vi "SEA-9510 FPGA.vi"() -> ()   [LabVIEW 2019]
doc: "Copyright (c) 2015-2019 S.E.A. Datentechnik GmbH, Germany"
uses:
  <vilib>/rvi/Emulation/niFpgaSctlEmulationGetInTimedLoop.vi
  <vilib>/rvi/Emulation/niFpgaProcessEmulError.vi
  <vilib>/rvi/eio/common/nirviEmuTemplateMethod_errors.vi
  <vilib>/rvi/Emulation/niFpgaGetClockAttributes.vi
  <vilib>/rvi/Emulation/niFpgaEmulationReportErrorSimple.vi
  <vilib>/rvi/Emulation/niFpgaCriticalErrorInLSC.vi
  <vilib>/eio/EIOMethodNode/EIOMethodNode.xnode
  <vilib>/eio/EIONode/EIONode.xnode
panel:
  in  "Numeric 3":i16
  out "Numeric 2":i16
  in  "Boolean":bool
  out "Numeric":i16
  out "Mod1/Ch3 Status":u16 format="%b"
  out "Mod1/Ch3 Add Info1":u16
  out "Mod1/Ch2 Status":u16 format="%b"
  out "Mod1/Ch2 Add Info1":u16
  out "Mod1/Ch1 Status":u16 format="%b"
  out "Mod1/Ch1 Add Info1":u16
  out "Mod1/Ch3 Abs Pos":u64
  out "Mod1/Ch2 Abs Pos":u64 format="%0d"
  out "Mod1/Ch1 Abs Pos":u64 format="%0.0f"
  out "Encoder Warnings":cluster{"Ch1":u16, "Ch2":u16, "Ch3":u16}
  out "Encoder Errors":cluster{"Ch1":u16, "Ch2":u16, "Ch3":u16}
  in  "Bus Speed":T1(ring)=enum."1 MHz"
  out "Initialized":bool
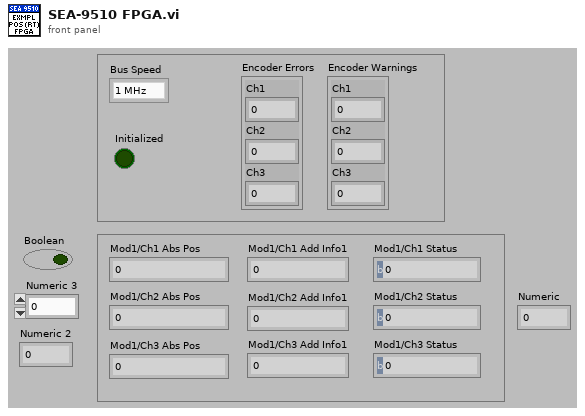
[diagram p1: front panel]
types:
  T1 = enum8{"8 MHz", "4 MHz", "2 MHz", "1 MHz", "200 kHz", "100 kHz"}
  T2 = enum8{"NOP", "Diagnosis", "Abs. Position Value 1 (LSB)", "Abs. Position Value 2", "Abs. Position Value 3 (MSB)", "Ackn. Memory Param. (LSB)", "Ackn. Memory Param. (MSB)", "Acknowledge MRS code", "Ackn. Test Command", "Send Test Value 1 (LSB)", "Send Test Value 2", "Send Test Value 3 (MSB)", "Temperature Sensor1", "Temperature Sensor2", "Addtl. Sensors", "Stop Sending Info1"}
  T3 = enum8{"NOP", "Commutation", "Acceleration", "Commut. & Acceler.", "Marginality Signal", "Marginality & Acceler.", "Asynchr. Pos Value 1 (LSB)", "Asynchr. Pos Value 2", "Asynchr. Pos Value 3 (MSB)", "Operating State Error", "Unused", "timestamp", "Reserved1", "Reserved2", "Reserved3", "Stop Sending Info2"}
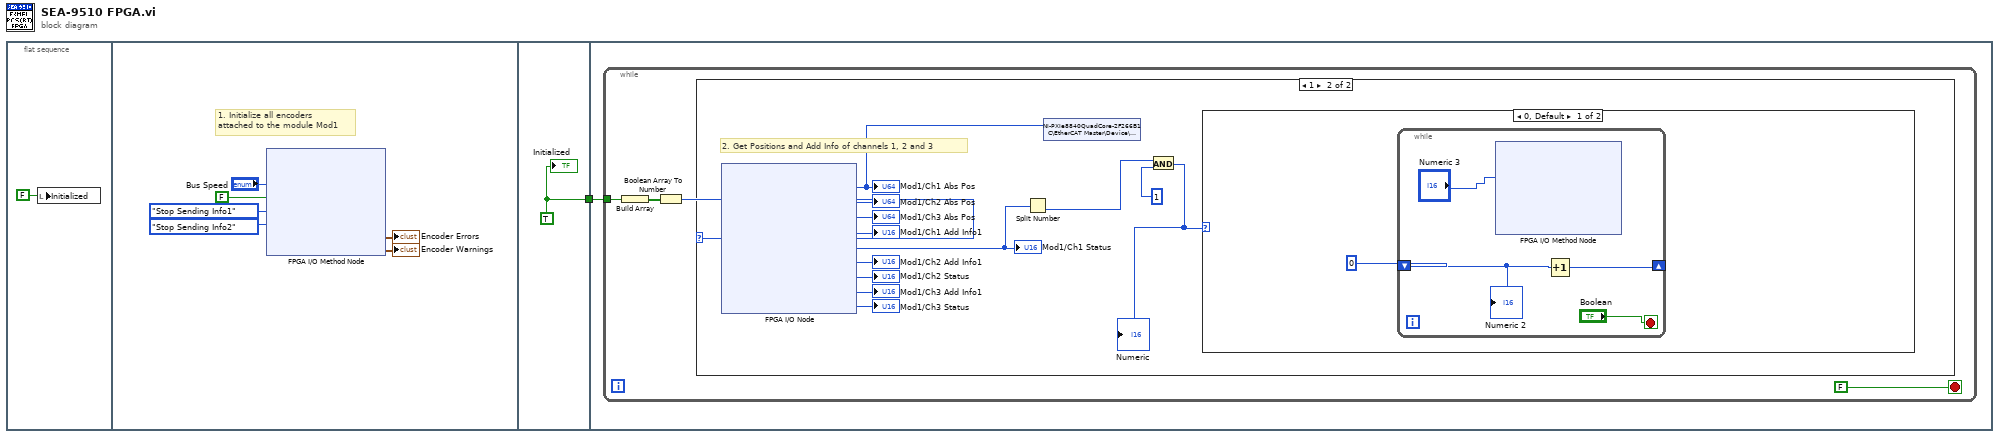
[diagram p0: block diagram]
diagram:
  n1 = flat-sequence {
    tunnel: [w9] -> w1
    tunnel: w1 -> [w10]
    frame #0 {
      n2 = local write "Initialized"(FALSE ("Initialized")) -> ()
    }
    frame #1 {
      # "1. Initialize all encoders\nattached to the module Mod1"
      n3 = xnode "FPGA I/O Method Node"("Bus Speed"="Bus Speed", "Enable Add Info"=FALSE, "Add Info1"=T2."Stop Sending Info1", "Add Info2"=T3."Stop Sending Info2") -> ("Encoder Errors"=→"Encoder Errors":cluster{"Ch1":u16, "Ch2":u16, "Ch3":u16}, "Encoder Warnings"=→"Encoder Warnings":cluster{"Ch1":u16, "Ch2":u16, "Ch3":u16})  [unwired: 1 in, 1 out]
    }
    frame #2 {
      w9 = TRUE ("Initialized")
      "Initialized" <- w9
    }
    frame #3 {
      n4 = while {
        tunnel: w10 -> [w12]
        stop <- FALSE stop-if-true
        n5 = Build Array(w12) -> (w13:bool[])
        n6 = Boolean Array To Number(Boolean array=w13) -> (number=w11:u8)
        n7 = case shown="1" w11 {
          frame 0, Default {
          }
          frame 1 {
            # "2. Get Positions and Add Info of channels 1, 2 and 3"
            n8 = xnode "FPGA I/O Node"() -> ("Mod1/Ch1 Abs Pos"=w15:u64, "Mod1/Ch2 Abs Pos"=→"Mod1/Ch2 Abs Pos":u64, "Mod1/Ch3 Abs Pos"=→"Mod1/Ch3 Abs Pos":u64, "Mod1/Ch1 Add Info1"=→"Mod1/Ch1 Add Info1":u16, "Mod1/Ch1 Status"=w19:u16, "Mod1/Ch2 Add Info1"=→"Mod1/Ch2 Add Info1":u16, "Mod1/Ch2 Status"=→"Mod1/Ch2 Status":u16, "Mod1/Ch3 Add Info1"=→"Mod1/Ch3 Add Info1":u16, "Mod1/Ch3 Status"=→"Mod1/Ch3 Status":u16)  [unwired: 9 in, 9 out]
            "Mod1/Ch1 Abs Pos" <- w15
            "Mod1/Ch1 Status" <- w19
            n9 = Split Number(x=w19) -> (lo(x)=w18:u8)  [unwired: 1 out]
            n10 = shared-variable "NI-PXIe8840QuadCore-2F266B1C\\EtherCAT Master\\Device\\User-Defined Variables\\Ch1 Position"(w15) -> ()  [unwired: 1 in, 1 out]
            n11 = And(x=w18, y=u8 1) -> (x .and. y?=w16:u8)
            "Numeric" <- w16
            n12 = case shown="0, Default" w16 {
              frame 0, Default {
                n13 = while {
                  shift-right: [w29] -> _
                  shift-left: i16 0 -> [w30]
                  stop <- "Boolean" stop-if-true
                  n14 = xnode "FPGA I/O Method Node"("Timeout"="Numeric 3") -> ()  [unwired: 1 in, 5 out]
                  n15 = Increment(x=w30) -> (x+1=w29:i16)
                  "Numeric 2" <- w30
                }
              }
              frame 1 {
              }
            }
          }
        }
      }
    }
  }
